vi "send_internal_trigger.vi"(8 "error in (no error)":errorcluster, 10 "trigger":T1, 11 "ScanHeadAK130114ResonanceFlexRIO in":refnum<class "ScanHeadAK130114ResonanceFlexRIO.lvclass">) -> (0 "error out":errorcluster, 3 "ScanHeadAK130114ResonanceFlexRIO out":refnum<class "ScanHeadAK130114ResonanceFlexRIO.lvclass">)   [LabVIEW 2010, in "ScanHeadAK130114ResonanceFlexRIO.lvclass"]
uses:
  ScanHeadAK130114ResonanceFlexRIO.lvclass
  ScanHeadMH100729FPGA/ScanHeadMH100729FPGA/internal_trigger_enum.ctl
  common/classes/GenericToplevelComponent/GenericToplevelComponent/trigger_type_enum.ctl
  ScanHeadMH100729FPGA/ScanHeadMH100729FPGA/ScanHeadMH100729FPGA.lvclass
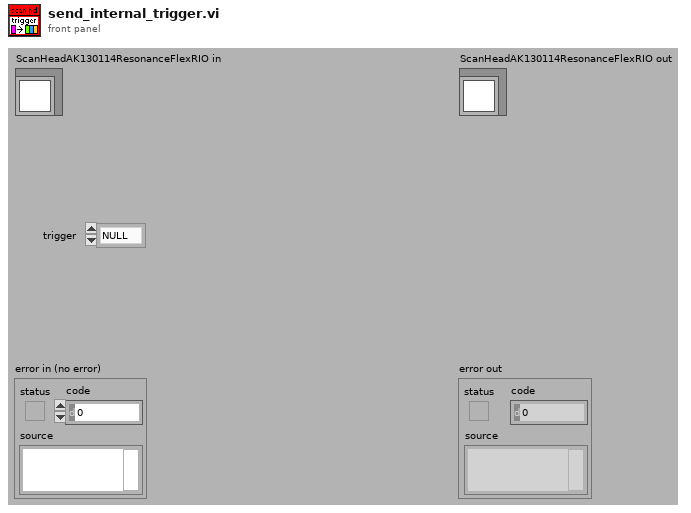
[diagram p1: front panel]
types:
  T1 = typedef "ScanHeadMH100729FPGA.lvclass/internal_trigger_enum.ctl" = enum16{"NULL", "initialise", "terminate", "start scanning", "stop scanning", "update", "fetch trajectory", "update bounding box"}
  T2 = typedef "trigger_type_enum.ctl" = enum8{"external", "internal", "common"}
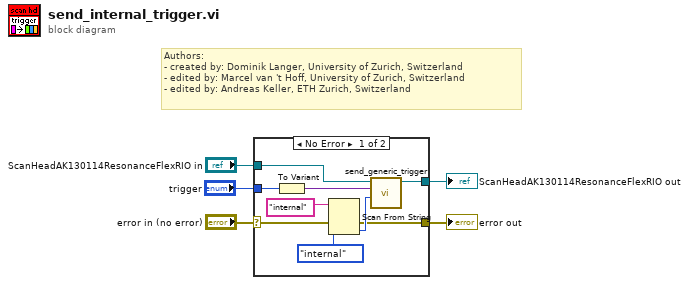
[diagram p0: block diagram]
diagram:
  # "Authors: \n- created by: Dominik Langer, University of Zurich, Switzerland\n- edited by: Marcel van 't Hoff, University of Zurich, Switzerland\n- edited by: Andreas Keller, ETH Zurich, Switzerland"
  n1 = case shown="No Error" "error in (no error)" {
    selector: "error in (no error)" -> [w10 w16]
    tunnel: [w9 w16] -> w4
    tunnel: [w13 w15] -> w2
    tunnel: "ScanHeadAK130114ResonanceFlexRIO in" -> [w14 w15]
    tunnel: "trigger" -> [w7 _]
    frame No Error {
      n2 = To Variant(anything=w7) -> (Variant=w6:variant)
      n3 = Scan From String(input string="internal", error in=w10, default 1=trigger_type_enum."internal" ("trigger type")) -> (error out=w9:errorcluster, output 1=w12:T2)  [unwired: 2 in, 2 out]
      n4 = call-dynamic "send_generic_trigger.vi"("trigger type"=w12, "trigger variant"=w6, "GenericToplevelComponent in"=w14) -> ("GenericToplevelComponent out"=w13:refnum<class "ScanHeadAK130114ResonanceFlexRIO.lvclass">)  [unwired: 5 in, 3 out]
    }
    frame Error {
    }
  }
  "error out" <- w4
  "ScanHeadAK130114ResonanceFlexRIO out" <- w2
